vi "HTTP POST XML Data.vi"(5 "webService/path (api)":string="api", 7 "port (80)":u16=80, 8 "error in (no error)":errorcluster, 9 "Timeout ms (30000)":i32=30000, 10 "XML Content":string, 11 "address (localhost)":string="localhost") -> (0 "error out":errorcluster, 1 "Timeout?":bool, 2 "XML Response":string, 3 "Comm Loop Time":u32)   [LabVIEW 2011]
panel:
  out "Max Loop Time":u32 caption="Max"
  out "Avg Loop Time":dbl caption="Avg"
  out "Time to read response":u32
  # "http://"
  # ":"
  # "/"
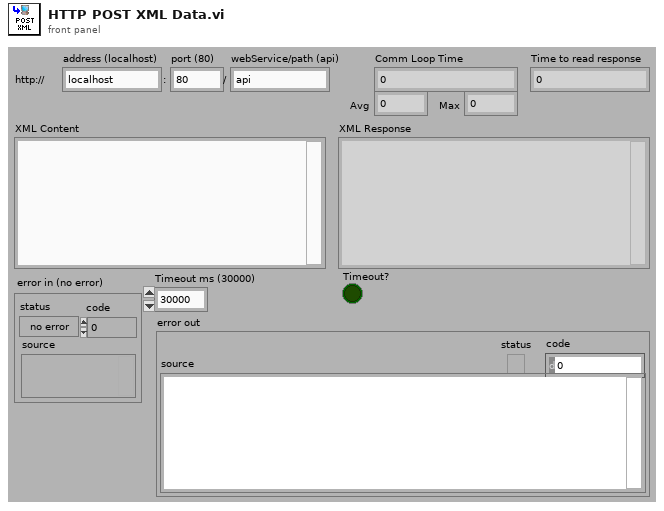
[diagram p1: front panel]
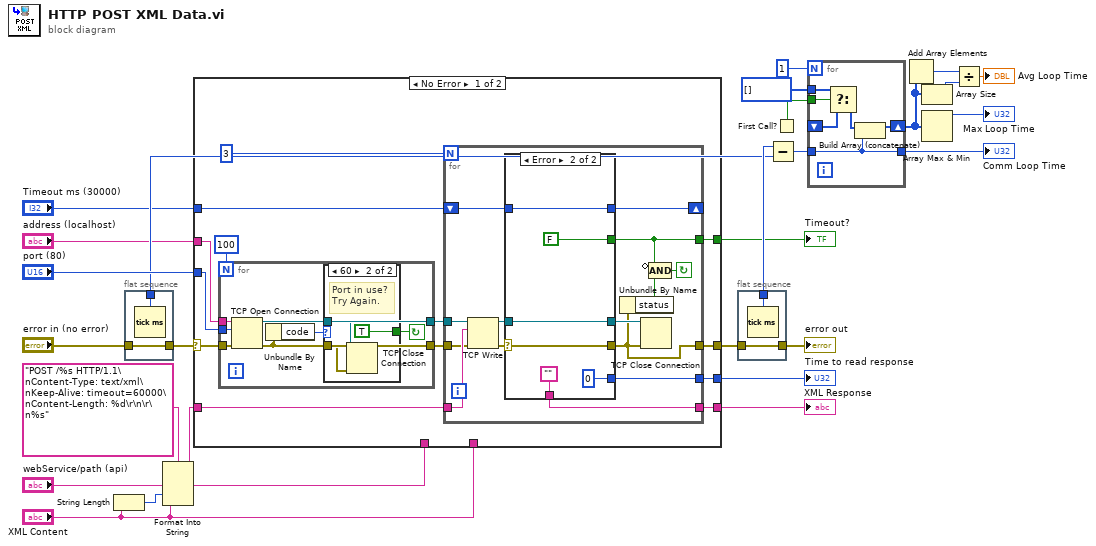
[diagram p0: block diagram]
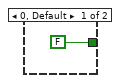
[diagram p2: hidden frame]
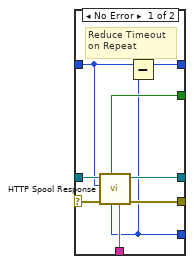
[diagram p3: hidden frame]
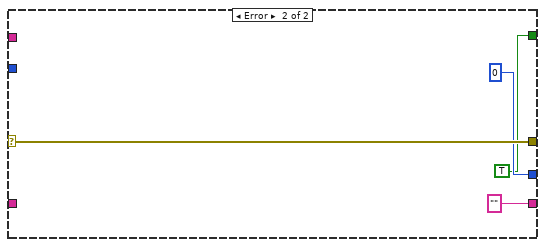
[diagram p4: hidden frame]
diagram:
  n1 = String Length(string="XML Content") -> (length=w25:i32)
  n2 = flat-sequence {
    tunnel: "error in (no error)" -> [w29]
    tunnel: [w29] -> w14
    tunnel: [w28] -> w18
    frame #0 {
      n3 = Tick Count (ms)() -> (millisecond timer value=w28:u32)
    }
  }
  n4 = Format Into String(format string="POST /%s HTTP/1.1\nContent-Type: text/xml\nKeep-Alive: timeout=60000\nContent-Length: %d\r\n\r\n%s" ("header"), "webService/path (api)", w25, "XML Content") -> (resulting string=w24:string)  [unwired: 2 in, 1 out]
  n5 = case shown="No Error" w14 {
    selector: w14 -> [w34 w86]
    tunnel: "port (80)" -> [w35 _]
    tunnel: w24 -> [w42 _]
    tunnel: [w41 "" ("RESPONSE Content Only")] -> w23
    tunnel: [w38 w86] -> w21
    tunnel: "address (localhost)" -> [w36 _]
    tunnel: [w40 u32 0 ("Time to receive response")] -> w16
    tunnel: "Timeout ms (30000)" -> [w39 _]
    tunnel: [w37 TRUE] -> w3
    tunnel: "webService/path (api)" -> [_ _]
    tunnel: "XML Content" -> [_ _]
    frame No Error {
      n6 = for {
        N: 100 -> [_]
        tunnel: w36 -> [w49]
        tunnel: w35 -> [w48]
        tunnel: w34 -> [w47]
        tunnel: [w44] -> w33
        tunnel: [w43] -> w32
        stop <- w45 continue-if-true
        n7 = TCP Open Connection(address=w49, remote port or service name=w48, error in (no error)=w47) -> (connection ID=w43:refnum<k5>, error out=w44:errorcluster)  [unwired: 2 in]
        n8 = Unbundle By Name(w44) -> ("code"=w46:i32)
        n9 = case shown="60" w46 {
          tunnel: [FALSE TRUE] -> w45
          tunnel: w44 -> [_ w52]
          tunnel: w43 -> [_ w51]
          frame 0, Default {
          }
          frame 60 {
            # "Port in use?\nTry Again."
            n10 = TCP Close Connection(connection ID=w51, error in (no error)=w52) -> ()  [unwired: 1 in, 2 out]
          }
        }
      }
      n11 = for {
        N: 3 -> [_]
        tunnel: w42 -> [w67]
        tunnel: [w66] -> w41
        tunnel: [w65] -> w40
        tunnel: [w56] -> w38
        tunnel: [w59] -> w37
        shift-right: [w57] -> _
        shift-left: w39 -> [w64]
        tunnel: w33 -> [w55]
        tunnel: w32 -> [w54]
        stop <- w58 continue-if-true
        n12 = TCP Write(connection ID=w54, data in=w67, error in (no error)=w55) -> (connection ID out=w62:refnum<k5>, error out=w63:errorcluster)  [unwired: 1 in, 1 out]
        n13 = case shown="Error" w63 {
          selector: w63 -> [w75 w81]
          tunnel: [w72 ""] -> w66
          tunnel: [w76 w81] -> w56
          tunnel: w62 -> [w74 w79]
          tunnel: [w73 w79] -> w61
          tunnel: [w69 u32 0 ("Time to receive response")] -> w65
          tunnel: w64 -> [w70 w77]
          tunnel: [w71 FALSE] -> w59
          tunnel: [w68 w77] -> w57
          frame No Error {
            # "Reduce Timeout\non Repeat"
            n14 = call "HTTP Spool Response.vi"("error in (no error)"=w75, "Timeout (ms)"=w70, "connection ID"=w74) -> ("error out"=w76:errorcluster, "connection ID out"=w73:refnum<k5>, "HTTP Body"=w72:string, "Time to receive response"=w69:u32, "timeout expired?"=w71:bool)  [unwired: 1 in, 3 out]
            n15 = Subtract(x=w70, y=w69) -> (x-y=w68:u32)
          }
          frame Error {
          }
        }
        n16 = Unbundle By Name(w56) -> ("status"=w60:bool)
        n17 = TCP Close Connection(connection ID=w61, error in (no error)=w56) -> ()  [unwired: 1 in, 2 out]
        n18 = Compound Arithmetic op=AND(invert w59, w60) -> (w58:bool)
      }
    }
    frame Error {
    }
  }
  "XML Response" <- w23
  "Time to read response" <- w16
  "Timeout?" <- w3
  n19 = flat-sequence {
    tunnel: w21 -> [w88]
    tunnel: [w88] -> w20
    tunnel: [w87] -> w19
    frame #0 {
      n20 = Tick Count (ms)() -> (millisecond timer value=w87:u32)
    }
  }
  n21 = Subtract(x=w19, y=w18) -> (x-y=w12:u32)
  n22 = First Call?() -> (First Call?: T/F=w5:bool)
  n23 = for {
    N: 1 -> [_]
    tunnel: w12 -> [w89]
    shift-right: [w94] -> w8
    shift-left: _ -> [w91]
    tunnel: u32[] [] -> [w92]
    tunnel: w5 -> [w90]
    tunnel: [w89] -> w4
    n24 = Select(t=w92, s=w90, f=w91) -> (s? t:f=w93:u32[])
    n25 = Build Array (concatenate)(w93, w89) -> (w94:u32[])
  }
  "Comm Loop Time" <- w4
  n26 = Add Array Elements(numeric array=w8) -> (sum=w10:u32)
  n27 = Array Size(array=w8) -> (size(s)=w11:i32)
  n28 = Array Max & Min(array=w8) -> (max value=→"Max Loop Time":u32)  [unwired: 3 out]
  n29 = Divide(x=w10, y=w11) -> (x/y=→"Avg Loop Time":dbl)
  "error out" <- w20
